vi "Initialize and Finalize.vi"(8 "error in (no error)":errorcluster) -> (0 "error out":errorcluster)   [LabVIEW 2020]
uses:
  G-Embedded-Python-Interpreter-Toolkit/Merge Call Library Errors.vi
  <vilib>/addons/_JKI Toolkits/Caraya/classes/Assert/Assert False.vi
  <vilib>/addons/_JKI Toolkits/Caraya/classes/Assert/Assert Not Error.vi
  <vilib>/addons/_JKI Toolkits/Caraya/classes/Assert/Assert True.vi
  G-Embedded-Python-Interpreter-Toolkit/G-Embedded-Python-Interpreter-Toolkit.lvlib
  <vilib>/addons/_JKI Toolkits/Caraya/classes/Assert/Assert.lvclass
  <vilib>/addons/_JKI Toolkits/Caraya/classes/Test/Test.lvclass
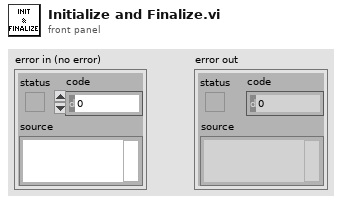
[diagram p1: front panel]
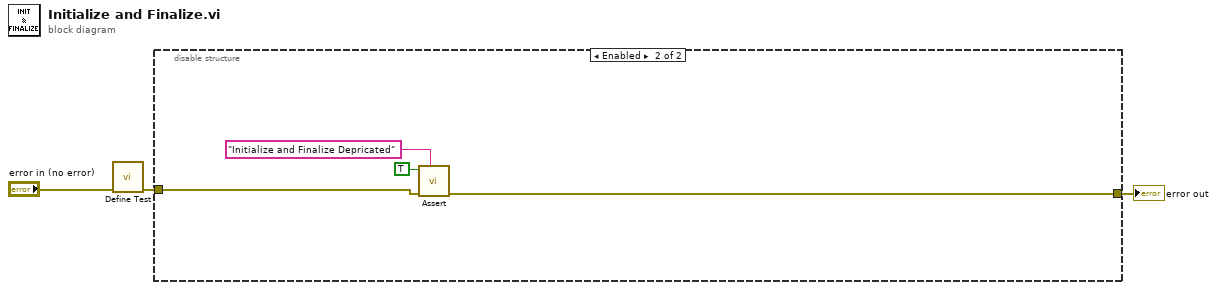
[diagram p0: block diagram]
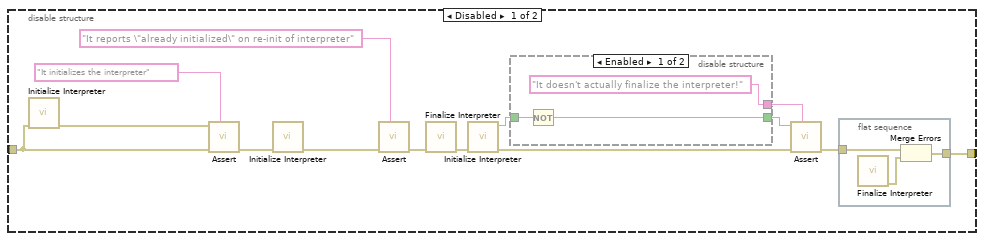
[diagram p2: hidden frame]
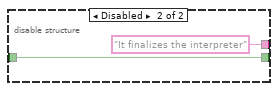
[diagram p3: hidden frame]
diagram:
  n1 = call <vilib>:"Define Test.vi"("error in (no error)"="error in (no error)") -> ("error out"=w3:errorcluster)  [unwired: 10 in]
  n2 = disable-structure shown="Enabled" {
    disable-tunnel: w3 -> [w16 w29]
    disable-tunnel: [w8 w28] -> w1
    frame Disabled {
      n3 = call "Initialize Interpreter.vi"("error in (no error)"=w16) -> ("error out"=w17:errorcluster)  [unwired: 9 in, 1 out]
      n4 = call-poly <vilib>:"Assert.vi"("Label"="It initializes the interpreter", "error in (no error)"=w16, "Not Error?"=w17) -> ("error out"=w14:errorcluster)  [unwired: 8 in]
      n5 = call "Initialize Interpreter.vi"("error in (no error)"=w14) -> ("error out"=w13:errorcluster)  [unwired: 9 in, 1 out]
      n6 = call-poly <vilib>:"Assert.vi"("Label"="It reports \"already initialized\" on re-init of interpreter", "error in (no error)"=w13) -> ("error out"=w11:errorcluster)  [unwired: 9 in]
      n7 = call "Finalize Interpreter.vi"("error in (no error)"=w11) -> ("error out"=w10:errorcluster)  [unwired: 10 in]
      n8 = call "Initialize Interpreter.vi"("error in (no error)"=w10) -> ("error out"=w9:errorcluster, "Already Initialized"=w5:bool)  [unwired: 9 in]
      n9 = disable-structure "Diagram Disable Structure" shown="Enabled" {
        disable-tunnel: [w18 w22] -> w6
        disable-tunnel: w5 -> [w19 w22]
        disable-tunnel: ["It doesn't actually finalize the interpreter!" ("Label") "It finalizes the interpreter" ("Label")] -> w4
        frame Enabled {
          n10 = Not(x=w19) -> (.not. x?=w18:bool)
        }
        frame Disabled {
        }
      }
      n11 = call-poly <vilib>:"Assert.vi"("Label"=w4, "error in (no error)"=w9, "False?"=w6) -> ("error out"=w7:errorcluster)  [unwired: 8 in]
      n12 = flat-sequence {
        tunnel: [w23] -> w8
        tunnel: w7 -> [w25]
        frame #0 {
          n13 = call "Finalize Interpreter.vi"() -> ("error out"=w24:errorcluster)  [unwired: 11 in]
          n14 = Merge Errors(w25, w24) -> (w23:errorcluster)
        }
      }
    }
    frame Enabled {
      n15 = call-poly <vilib>:"Assert.vi"("Label"="Initialize and Finalize Depricated", "error in (no error)"=w29, "True?"=TRUE) -> ("error out"=w28:errorcluster)  [unwired: 8 in]
    }
  }
  "error out" <- w1
